vi "CtrlTreeGetAppRef.vi"(8 "error in (no error)":errorcluster, 9 "App Tag":string, 11 "ControlTree in":refnum<vi>) -> (0 "error out":errorcluster, 1 "Path":string, 2 "Application out":refnum<vi>, 3 "ControlTree out":refnum<vi>)   [LabVIEW 2020]
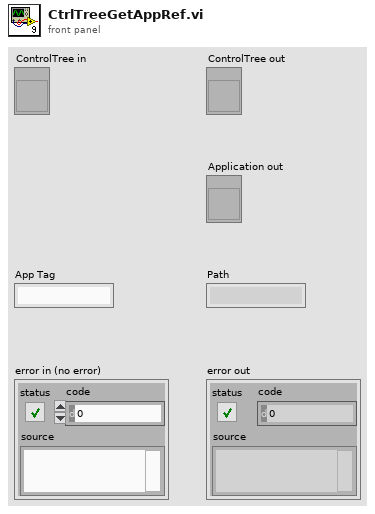
[diagram p1: front panel]
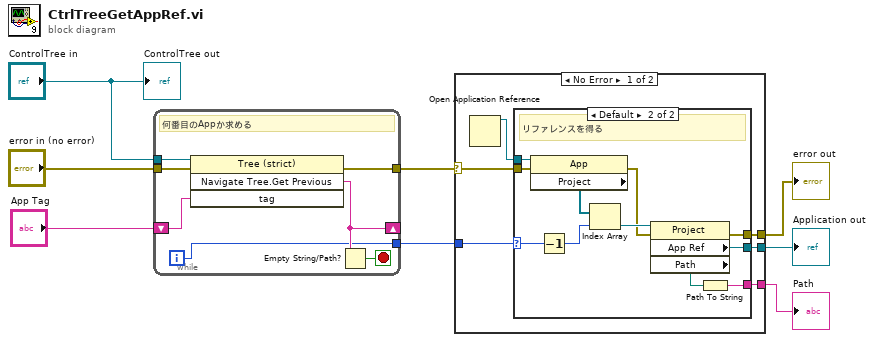
[diagram p0: block diagram]
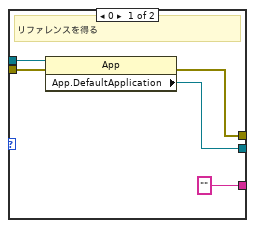
[diagram p2: hidden frame]
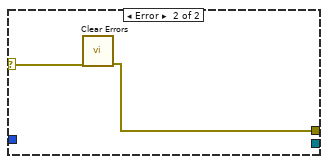
[diagram p3: hidden frame]
diagram:
  n1 = while {
    tunnel: "ControlTree in" -> [w15]
    shift-right: [w13] -> _
    shift-left: "App Tag" -> [w14]
    tunnel: [w11] -> w3
    tunnel: "error in (no error)" -> [w10]
    tunnel: [w9] -> w1
    i -> [w11]
    stop <- w12 stop-if-true
    # "何番目のAppか求める"
    n2 = invoke class="Tree (strict)" method="Navigate Tree.Get Previous"(reference=w15, error in=w10, "tag"=w14) -> (error out=w9:errorcluster, "Navigate Tree:Get Previous"=w13:string)  [unwired: 1 in, 2 out]
    n3 = Empty String/Path?(string/path=w13) -> (empty?=w12:bool)
  }
  n4 = case shown="No Error" w1 {
    selector: w1 -> [w16 w39]
    tunnel: [w21 w38] -> w8
    tunnel: [w20 _] -> w5
    tunnel: w3 -> [w19 _]
    tunnel: [w17 _] -> w2
    frame No Error {
      n5 = Open Application Reference() -> (3:w18:refnum<vi>)  [unwired: 4 in, 1 out]
      n6 = case shown="Default" w19 {
        selector: w19 -> [_ w36]
        tunnel: w18 -> [w26 w37]
        tunnel: [w25 w32] -> w20
        tunnel: w16 -> [w24 w31]
        tunnel: [w23 w29] -> w21
        tunnel: ["" w27] -> w17
        frame 0 {
          # "リファレンスを得る"
          n7 = property class="App"(reference=w26, error in=w24) -> (error out=w23:errorcluster, "App.DefaultApplication"=w25:refnum<vi>)  [unwired: 1 out]
        }
        frame Default {
          # "リファレンスを得る"
          n8 = property class="App"(reference=w37, error in=w31) -> (error out=w30:errorcluster, "Project"=w35:refnum<vi>[])  [unwired: 1 out]
          n9 = Decrement(x=w36) -> (x-1=w34:i32)
          n10 = Index Array(array=w35, index=w34) -> (element=w33:refnum<vi>)
          n11 = property class="Project"(reference=w33, error in=w30) -> (error out=w29:errorcluster, "App Ref"=w32:refnum<vi>, "Path"=w28:path)  [unwired: 1 out]
          n12 = Path To String(path=w28) -> (string=w27:string)
        }
      }
    }
    frame Error {
      n13 = call <vilib>:"Clear Errors.vi"("error in (no error)"=w39) -> ("error out"=w38:errorcluster)  [unwired: 5 in, 1 out]
    }
  }
  "error out" <- w8
  "Application out" <- w5
  "Path" <- w2
  "ControlTree out" <- "ControlTree in"
